vi "Controller Enable Filters.vi"(8 "error in":errorcluster, 11 "Enable Controller Filters":bool) -> (0 "error out":errorcluster)   [LabVIEW 2011, in "Controller VIs.lvlib"]
uses:
  Controller VIs.lvlib
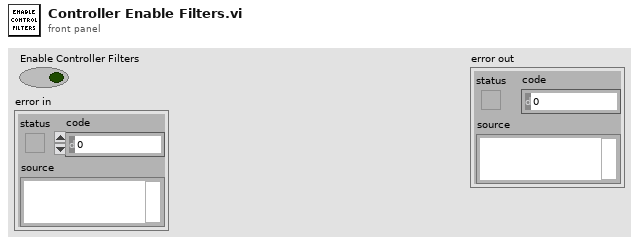
[diagram p1: front panel]
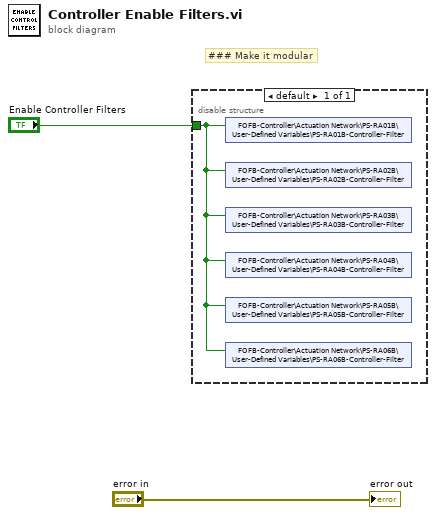
[diagram p0: block diagram]
diagram:
  # "### Make it modular"
  n1 = disable-structure shown="default" {
    disable-tunnel: "Enable Controller Filters" -> [w3]
    frame Enabled {
      n2 = shared-variable "FOFB-Controller\\Actuation Network\\PS-RA01B\\User-Defined Variables\\PS-RA01B-Controller-Filter"(w3) -> ()  [unwired: 1 in, 1 out]
      n3 = shared-variable "FOFB-Controller\\Actuation Network\\PS-RA02B\\User-Defined Variables\\PS-RA02B-Controller-Filter"(w3) -> ()  [unwired: 1 in, 1 out]
      n4 = shared-variable "FOFB-Controller\\Actuation Network\\PS-RA03B\\User-Defined Variables\\PS-RA03B-Controller-Filter"(w3) -> ()  [unwired: 1 in, 1 out]
      n5 = shared-variable "FOFB-Controller\\Actuation Network\\PS-RA04B\\User-Defined Variables\\PS-RA04B-Controller-Filter"(w3) -> ()  [unwired: 1 in, 1 out]
      n6 = shared-variable "FOFB-Controller\\Actuation Network\\PS-RA05B\\User-Defined Variables\\PS-RA05B-Controller-Filter"(w3) -> ()  [unwired: 1 in, 1 out]
      n7 = shared-variable "FOFB-Controller\\Actuation Network\\PS-RA06B\\User-Defined Variables\\PS-RA06B-Controller-Filter"(w3) -> ()  [unwired: 1 in, 1 out]
    }
  }
  "error out" <- "error in"
